vi "LedColorControl.vi"(7 "Button":bool) -> ()   [LabVIEW 2014]
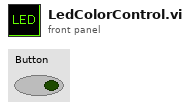
[diagram p1: front panel]
types:
  T1 = typedef "WPI_SPIDevRef.ctl" = cluster{"DevStatus":errorcluster, "Handle":i32, "Controller":T2, "SPI Bus":T3}
  T2 = typedef "FPGA_TypedefDigitalModule.ctl" = enum16{"Controller 1"}
  T3 = typedef "spi_bus.ctl" = enum16{"SPI On-Board, CS0", "SPI On-Board, CS1", "SPI On-Board, CS2", "SPI On-Board, CS3", "SPI MXP", "Invalid"}
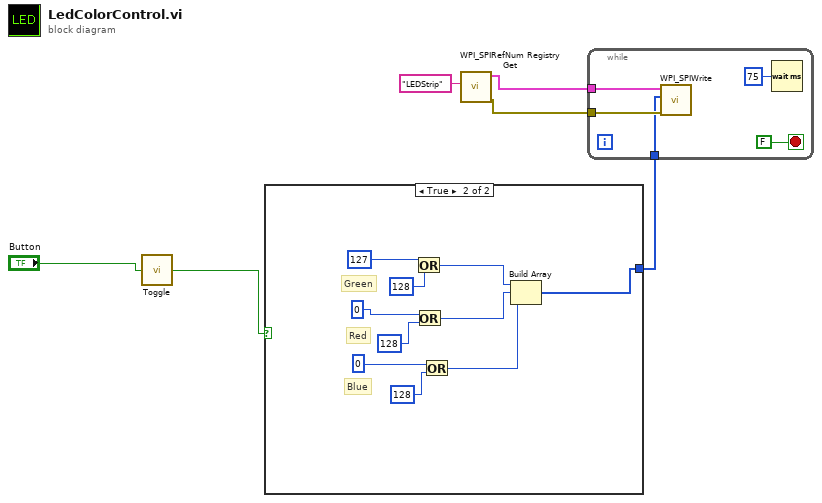
[diagram p0: block diagram]
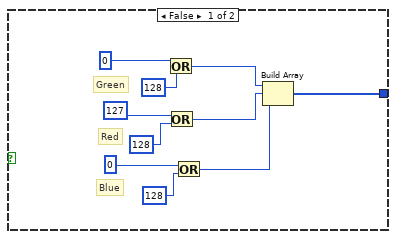
[diagram p2: hidden frame]
diagram:
  n1 = call "Toggle.vi"("Buton"="Button") -> ("Output"=w5:bool)
  n2 = case shown="True" w5 {
    tunnel: [w7 w17] -> w1
    frame False {
      # "Blue"
      # "Red"
      # "Green"
      n3 = Or(x=0, y=128) -> (x .or. y?=w10:i32)
      n4 = Or(x=127, y=128) -> (x .or. y?=w9:i32)
      n5 = Or(x=0, y=128) -> (x .or. y?=w8:i32)
      n6 = Build Array(w10, w9, w8) -> (w7:i32[])
    }
    frame True {
      # "Blue"
      # "Red"
      # "Green"
      n7 = Or(x=127, y=128) -> (x .or. y?=w20:i32)
      n8 = Or(x=0, y=128) -> (x .or. y?=w19:i32)
      n9 = Or(x=0, y=128) -> (x .or. y?=w18:i32)
      n10 = Build Array(w20, w19, w18) -> (w17:i32[])
    }
  }
  n11 = call <vilib>:"WPI_SPIRefNum Registry Get.vi"("refnum name"="LEDStrip") -> ("error out"=w2:errorcluster, "SPIDevRef"=w3:T1)  [unwired: 9 in]
  n12 = while {
    tunnel: w3 -> [w31]
    tunnel: w2 -> [w30]
    tunnel: w1 -> [w29]
    stop <- FALSE stop-if-true
    n13 = call <vilib>:"WPI_SPIWrite.vi"("error in (no error)"=w30, "Data To Send"=w29, "SPIDevRef"=w31) -> ()  [unwired: 6 in, 3 out]
    n14 = Wait (ms)(milliseconds to wait=u32 75) -> ()  [unwired: 1 out]
  }
